vi "SetHeaderVariantData.vi"(8 "error in (no error)":errorcluster, 9 "Value":string, 10 "Name":string, 11 "Variant in":variant) -> (0 "error out":errorcluster, 3 "Variant out":variant)   [LabVIEW 2013, in "WebSockets.lvlib"]
doc: "Sets a variant attribute. If the attribute already exists, it builds a comma separated string of the values (useful for keep array data)."
uses:
  WebSockets.lvlib
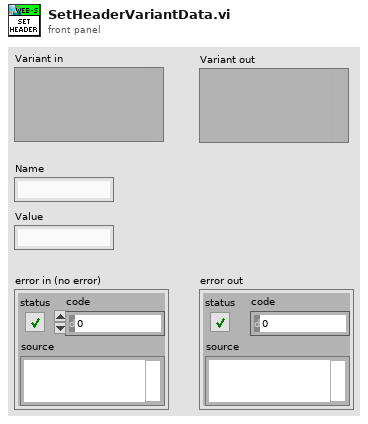
[diagram p1: front panel]
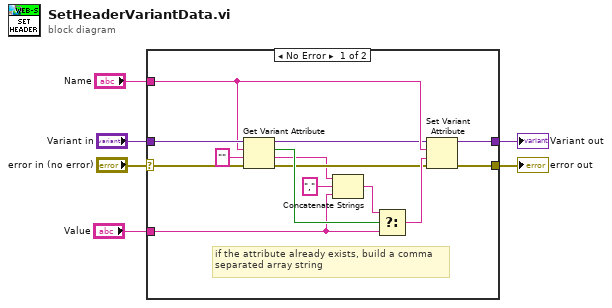
[diagram p0: block diagram]
diagram:
  n1 = case shown="No Error" "error in (no error)" {
    selector: "error in (no error)" -> [w7 w22]
    tunnel: [w20 w22] -> w6
    tunnel: [w19 w21] -> w5
    tunnel: "Variant in" -> [w18 w21]
    tunnel: "Name" -> [w17 _]
    tunnel: "Value" -> [w9 _]
    frame No Error {
      # "if the attribute already exists, build a comma\nseparated array string"
      n2 = Get Variant Attribute(Variant=w18, name=w17, default value (empty Variant)="", error in=w7) -> (duplicate Variant=w13:variant, found=w15:bool, value=w11:string, error out=w12:errorcluster)
      n3 = Concatenate Strings(w11, "," ("string"), w9) -> (w8:string)
      n4 = Select(t=w8, s=w15, f=w9) -> (s? t:f=w14:string)
      n5 = Set Variant Attribute(Variant=w13, name=w17, value=w14, error in=w12) -> (Variant out=w19:variant, error out=w20:errorcluster)  [unwired: 1 out]
    }
    frame Error {
    }
  }
  "error out" <- w6
  "Variant out" <- w5
